vi "Array of Zeros.vi"(8 "Index":T1={"N1"=18, "N2"=19, "N3"=4, "N4"=5, "V1"=8, "V2"=10, "V3"=10, "V4"=13, "CURRENT"=12, "Vsg"=1}, 9 "Single/Differential":bool=TRUE, 10 "Conductance":T2(graph), 11 "Folder Path":path) -> (3 "Conductance 2":T2(graph))   [LabVIEW 2016]
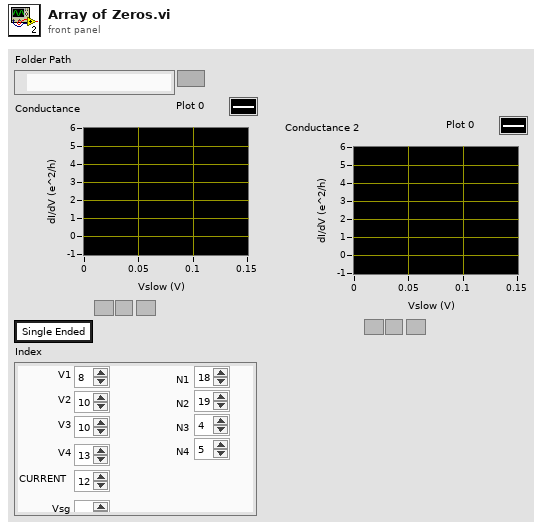
[diagram p1: front panel]
types:
  T1 = cluster{"N1":i32, "N2":i32, "N3":i32, "N4":i32, "V1":i32, "V2":i32, "V3":i32, "V4":i32, "CURRENT":i32, "Vsg":i32}
  T2 = cluster{"Vfast":dbl[], "Decimated Array":dbl[]}[]
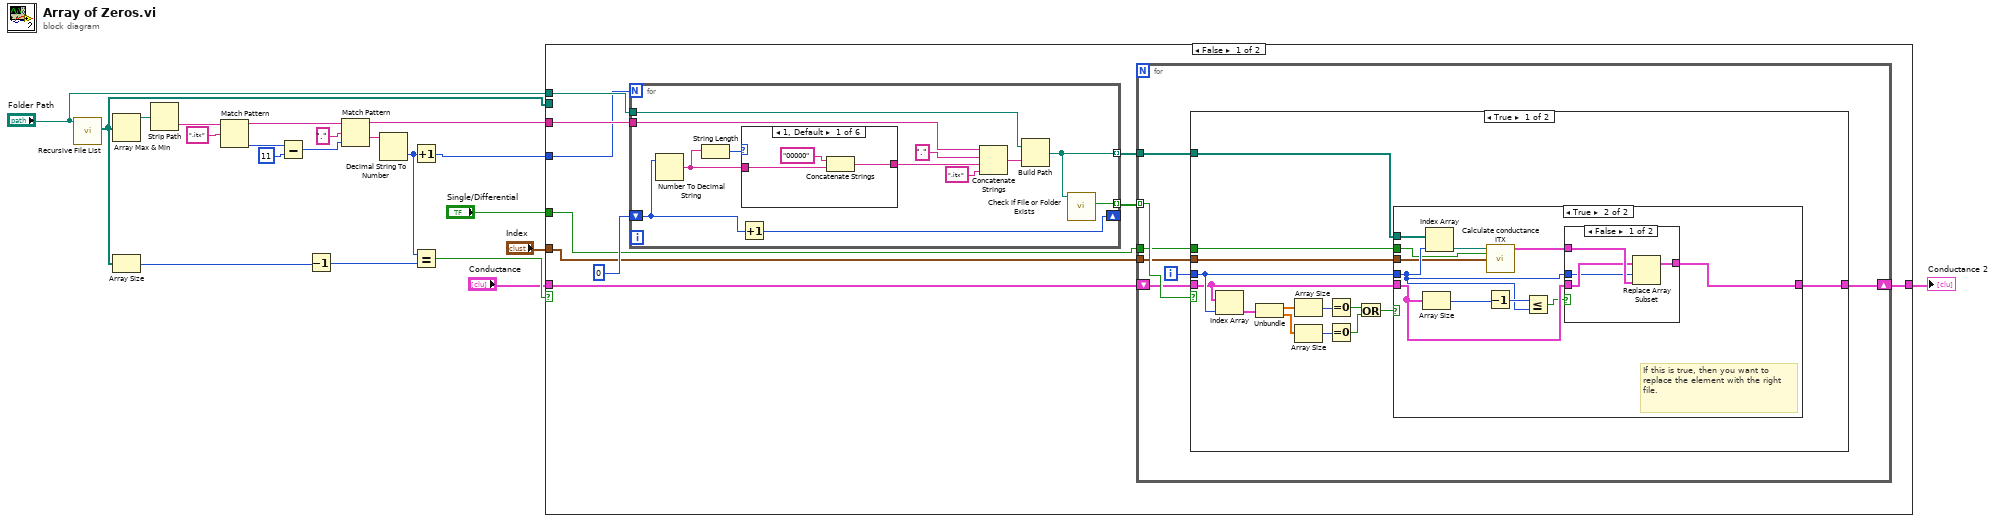
[diagram p0: block diagram]
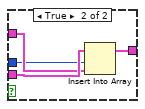
[diagram p3: hidden frame]
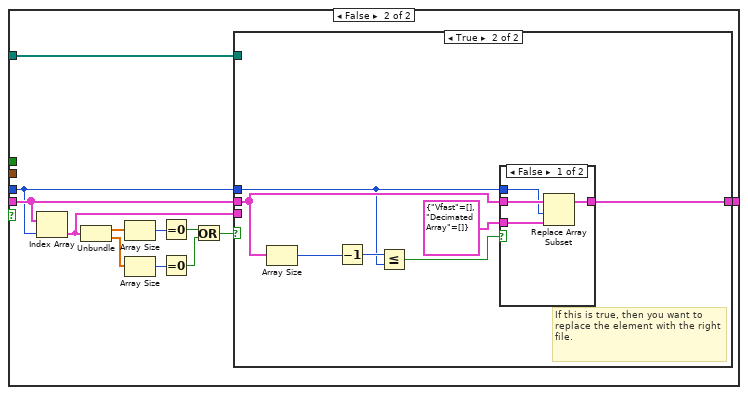
[diagram p4: hidden frame]
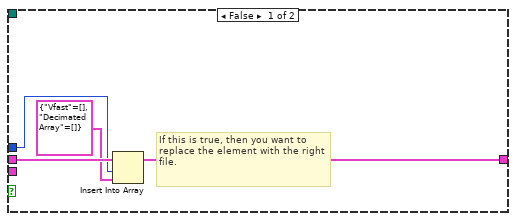
[diagram p5: hidden frame]
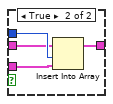
[diagram p6: hidden frame]
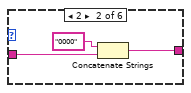
[diagram p7: hidden frame]
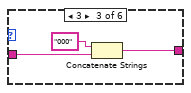
[diagram p8: hidden frame]
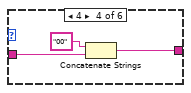
[diagram p9: hidden frame]
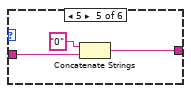
[diagram p10: hidden frame]
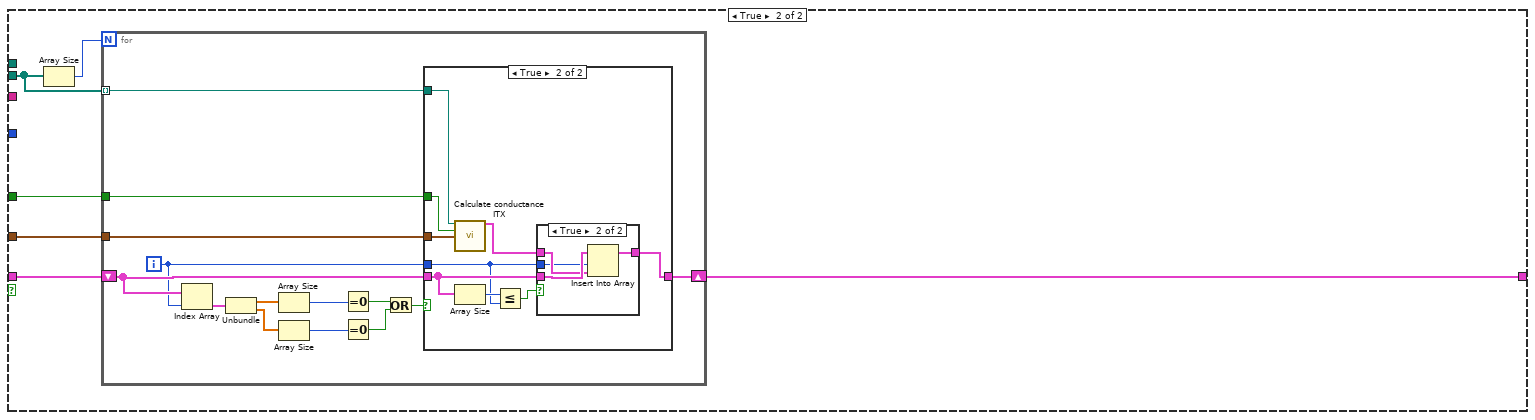
[diagram p12: hidden frame]
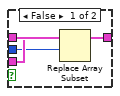
[diagram p14: hidden frame]
diagram:
  n1 = call <vilib>:"Recursive File List.vi"("Folder Path"="Folder Path") -> ("All Files in Dir"=w6:path[])  [unwired: 7 in, 3 out]
  n2 = Array Max & Min(array=w6) -> (max value=w13:path)  [unwired: 3 out]
  n3 = Array Size(array=w6) -> (size(s)=w12:i32)
  n4 = Strip Path(path=w13) -> (name=w21:string)  [unwired: 1 out]
  n5 = Match Pattern(string=w21, regular expression=".itx") -> (before substring=w16:string, offset past match=w19:i32)  [unwired: 1 in, 2 out]
  n6 = Subtract(x=w19, y=11) -> (x-y=w17:i32)
  n7 = Decrement(x=w12) -> (x-1=w11:i32)
  n8 = Match Pattern(string=w16, regular expression=".", offset (0)=w17) -> (before substring=w7:string, after substring=w14:string)  [unwired: 2 out]
  n9 = Decimal String To Number(string=w14) -> (number=w8:i32)  [unwired: 2 in, 1 out]
  n10 = Increment(x=w8) -> (x+1=w1:i32)
  n11 = Equal?(x=w8, y=w11) -> (x = y?=w10:bool)
  n12 = case shown="False" w10 {
    tunnel: "Folder Path" -> [w31 _]
    tunnel: w7 -> [w29 _]
    tunnel: "Conductance" -> [w25 w136]
    tunnel: [w26 w135] -> w4
    tunnel: w6 -> [_ w134]
    tunnel: "Single/Differential" -> [w24 w133]
    tunnel: "Index" -> [w23 w132]
    tunnel: w1 -> [w22 _]
    frame False {
      n13 = for {
        N: w22 -> [_]
        tunnel: w31 -> [w109]
        shift-right: [w106] -> _
        shift-left: 0 -> [w104]
        tunnel: w29 -> [w113]
        tunnel: [w107] -> w28 mode=indexing
        tunnel: [w105] -> w27 mode=indexing
        n14 = Number To Decimal String(number=w104) -> (decimal integer string=w115:string)  [unwired: 1 in]
        n15 = String Length(string=w115) -> (length=w114:i32)
        n16 = Increment(x=w104) -> (x+1=w106:i32)
        n17 = case shown="1, Default" w114 {
          tunnel: w115 -> [w117 w121 w124 w127 w130 w131]
          tunnel: [w116 w120 w122 w126 w129 w131] -> w111
          frame 1, Default {
            n18 = Concatenate Strings("00000" ("string"), w117) -> (w116:string)
          }
          frame 2 {
            n19 = Concatenate Strings("0000" ("string"), w121) -> (w120:string)
          }
          frame 3 {
            n20 = Concatenate Strings("000" ("string"), w124) -> (w122:string)
          }
          frame 4 {
            n21 = Concatenate Strings("00" ("string"), w127) -> (w126:string)
          }
          frame 5 {
            n22 = Concatenate Strings("0" ("string"), w130) -> (w129:string)
          }
          frame 6 {
          }
        }
        n23 = Concatenate Strings(w113, "." ("string"), w111, ".itx" ("string")) -> (w108:string)
        n24 = Build Path(base path=w109, name or relative path=w108) -> (appended path=w105:path)
        n25 = call <vilib>:"Check if File or Folder Exists.vi"("path"=w105) -> ("file or folder exists?"=w107:bool)  [unwired: 8 in, 2 out]
      }
      n26 = for {
        tunnel: w28 -> [w38] mode=indexing
        tunnel: w27 -> [w36]
        shift-right: [w35] -> w26
        shift-left: w25 -> [w34]
        tunnel: w24 -> [w33]
        tunnel: w23 -> [w32]
        i -> [w37]
        n27 = case shown="True" w38 {
          tunnel: w37 -> [w52 w83]
          tunnel: w34 -> [w49 w84]
          tunnel: w36 -> [w51 w82]
          tunnel: [w50 w81] -> w35
          tunnel: w33 -> [w40 _]
          tunnel: w32 -> [w39 _]
          frame True {
            n28 = Index Array(array=w49, index=w52) -> (element=w48:cluster{"Vfast":dbl[], "Decimated Array":dbl[]})
            n29 = Unbundle(w48) -> ("Vfast"=w47:dbl[], "Decimated Array"=w46:dbl[])
            n30 = Array Size(array=w47) -> (size(s)=w45:i32)
            n31 = Array Size(array=w46) -> (size(s)=w44:i32)
            n32 = Equal To 0?(x=w45) -> (x = 0?=w43:bool)
            n33 = Equal To 0?(x=w44) -> (x = 0?=w42:bool)
            n34 = Or(x=w43, y=w42) -> (x .or. y?=w41:bool)
            n35 = case shown="True" w41 {
              tunnel: w49 -> [w53 w61]
              tunnel: w52 -> [_ w58]
              tunnel: w51 -> [_ w64]
              tunnel: [w53 w56] -> w50
              tunnel: w40 -> [_ w55]
              tunnel: w39 -> [_ w54]
              frame False {
              }
              frame True {
                # "If this is true, then you want to replace the element with the right file."
                n36 = Array Size(array=w61) -> (size(s)=w60:i32)
                n37 = Index Array(array=w64, index=w58) -> (element=w63:path)
                n38 = Decrement(x=w60) -> (x-1=w59:i32)
                n39 = call "Calculate conductance ITX.vi"("File or Folder Path"=w63, "single ended?"=w55, "index"=w54) -> ("A vs D"=w62:cluster{dbl[], dbl[]}[])  [unwired: 9 in, 3 out]
                n40 = Less Or Equal?(x=w59, y=w58) -> (x <= y?=w57:bool)
                n41 = case shown="False" w57 {
                  tunnel: w62 -> [w68 w71]
                  tunnel: [w67 w69] -> w56
                  tunnel: w61 -> [w66 w72]
                  tunnel: w58 -> [w65 w70]
                  frame False {
                    n42 = Replace Array Subset(array=w66, new element=w68, index=w65) -> (w67:T2)
                  }
                  frame True {
                    n43 = Insert Into Array(array=w72, index=w70, new element=w71) -> (w69:T2)
                  }
                }
              }
            }
          }
          frame False {
            n44 = Index Array(array=w84, index=w83) -> (element=w74:cluster{"Vfast":dbl[], "Decimated Array":dbl[]})
            n45 = Unbundle(w74) -> ("Vfast"=w80:dbl[], "Decimated Array"=w79:dbl[])
            n46 = Array Size(array=w80) -> (size(s)=w78:i32)
            n47 = Array Size(array=w79) -> (size(s)=w77:i32)
            n48 = Equal To 0?(x=w78) -> (x = 0?=w76:bool)
            n49 = Equal To 0?(x=w77) -> (x = 0?=w75:bool)
            n50 = Or(x=w76, y=w75) -> (x .or. y?=w73:bool)
            n51 = case shown="True" w73 {
              tunnel: w84 -> [w88 w90]
              tunnel: w83 -> [w87 w89]
              tunnel: w82 -> [_ _]
              tunnel: [w86 w95] -> w81
              tunnel: w74 -> [_ _]
              frame False {
                # "If this is true, then you want to replace the element with the right file."
                n52 = Insert Into Array(array=w88, index=w87, new element=cluster{"Vfast":dbl[], "Decimated Array":dbl[]} {"Vfast"=[], "Decimated Array"=[]} ("x")) -> (w86:T2)
              }
              frame True {
                # "If this is true, then you want to replace the element with the right file."
                n53 = Array Size(array=w90) -> (size(s)=w93:i32)
                n54 = Decrement(x=w93) -> (x-1=w92:i32)
                n55 = Less Or Equal?(x=w92, y=w89) -> (x <= y?=w91:bool)
                n56 = case shown="False" w91 {
                  tunnel: w89 -> [w98 w103]
                  tunnel: [w96 w102] -> w95
                  tunnel: cluster{"Vfast":dbl[], "Decimated Array":dbl[]} {"Vfast"=[], "Decimated Array"=[]} ("x") -> [w97 w101]
                  tunnel: w90 -> [w99 w100]
                  frame False {
                    n57 = Replace Array Subset(array=w99, new element=w97, index=w98) -> (w96:T2)
                  }
                  frame True {
                    n58 = Insert Into Array(array=w100, index=w103, new element=w101) -> (w102:T2)
                  }
                }
              }
            }
          }
        }
      }
    }
    frame True {
      n59 = Array Size(array=w134) -> (size(s)=w137:i32)
      n60 = for {
        N: w137 -> [_]
        shift-right: [w140] -> w135
        shift-left: w136 -> [w143]
        tunnel: w134 -> [w142] mode=indexing
        tunnel: w133 -> [w139]
        tunnel: w132 -> [w138]
        i -> [w141]
        n61 = Index Array(array=w143, index=w141) -> (element=w145:cluster{"Vfast":dbl[], "Decimated Array":dbl[]})
        n62 = Unbundle(w145) -> ("Vfast"=w151:dbl[], "Decimated Array"=w150:dbl[])
        n63 = Array Size(array=w151) -> (size(s)=w149:i32)
        n64 = Array Size(array=w150) -> (size(s)=w148:i32)
        n65 = Equal To 0?(x=w149) -> (x = 0?=w147:bool)
        n66 = Equal To 0?(x=w148) -> (x = 0?=w146:bool)
        n67 = Or(x=w147, y=w146) -> (x .or. y?=w144:bool)
        n68 = case shown="True" w144 {
          tunnel: w143 -> [w152 w158]
          tunnel: w142 -> [_ w161]
          tunnel: w141 -> [_ w156]
          tunnel: [w152 w159] -> w140
          tunnel: w139 -> [_ w154]
          tunnel: w138 -> [_ w153]
          frame False {
          }
          frame True {
            n69 = call "Calculate conductance ITX.vi"("File or Folder Path"=w161, "single ended?"=w154, "index"=w153) -> ("A vs D"=w160:cluster{dbl[], dbl[]}[])  [unwired: 9 in, 3 out]
            n70 = Array Size(array=w158) -> (size(s)=w157:i32)
            n71 = Less Or Equal?(x=w157, y=w156) -> (x <= y?=w155:bool)
            n72 = case shown="True" w155 {
              tunnel: w160 -> [w165 w168]
              tunnel: [w164 w166] -> w159
              tunnel: w158 -> [w163 w169]
              tunnel: w156 -> [w162 w167]
              frame False {
                n73 = Replace Array Subset(array=w163, new element=w165, index=w162) -> (w164:T2)
              }
              frame True {
                n74 = Insert Into Array(array=w169, index=w167, new element=w168) -> (w166:T2)
              }
            }
          }
        }
      }
    }
  }
  "Conductance 2" <- w4
